vi "FormatCrvNames.vi"(8 "entrée d'erreur":errorcluster, 11 "CurveNamesIn":string[](array[string])) -> (0 "sortie d'erreur":errorcluster, 3 "CurveNames":string[](array[string]))   [LabVIEW 2019]
doc: "Ce Vi prend le tableau des noms de courbe au format Scanlist et retire la partie \"_Scan|Log\". La partie retiré correspond au caractère \"_\" suivi du préfixe de scan ou de log spécifié dans Labscan.ini. Pour les scan à plusieurs ordres, la partie spécifiant l'indice du paramètre de 2e ordre (ex: _par0) est remis en place.\nEx:\nTools.Temps Abs (ms)_Scan0 -> Tools.Temps Abs (ms)\nTools.Temps Abs (ms)_Scan0@Tools.Indice de Points(points)_par0 -> Tools.Temps Abs (ms)_par0"
uses:
  <vilib>/regexp/Match Regular Expression.xnode
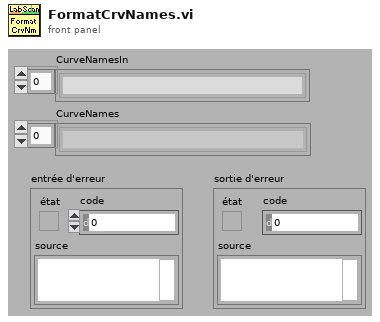
[diagram p1: front panel]
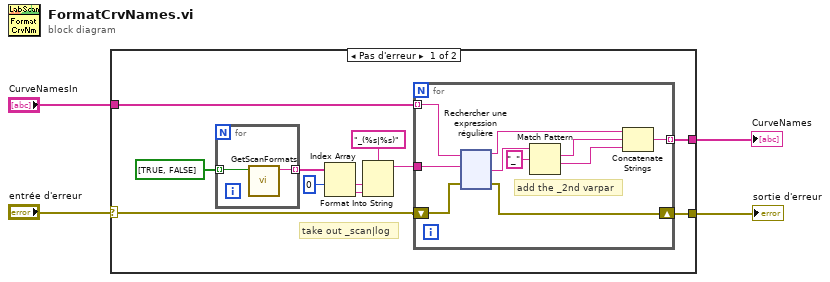
[diagram p0: block diagram]
diagram:
  n1 = case shown="Pas d'erreur" "entrée d'erreur" {
    selector: "entrée d'erreur" -> [w5 w139]
    tunnel: "CurveNamesIn" -> [w15 _]
    tunnel: [w7 _] -> w2
    tunnel: [w6 w139] -> w3
    frame No Error {
      # "take out _scan|log"
      n2 = for {
        tunnel: bool[] [TRUE, FALSE] -> [w138] mode=indexing
        tunnel: [w137] -> w13 mode=indexing
        n3 = call "GetScanFormats.vi"("Scan(T)"=w138) -> ("Prefixe"=w137:string)  [unwired: 8 in, 2 out]
      }
      n4 = Index Array(array=w13, index #1=0 ("indice")) -> (element #1=w10:string, element #2=w9:string)  [unwired: 1 in]
      n5 = Format Into String(format string="_(%s|%s)" ("chaîne de format"), w10, w9) -> (resulting string=w8:string)  [unwired: 2 in, 1 out]
      n6 = for {
        tunnel: w15 -> [w25] mode=indexing
        tunnel: w8 -> [w24]
        tunnel: [w20] -> w7 mode=indexing
        shift-right: [w17] -> w6
        shift-left: w5 -> [w16]
        # "add the _2nd varpar"
        n7 = xnode "Rechercher une expression régulière"("chaîne en entrée"=w25, "expression régulière"=w24, "entrée d'erreur"=w16) -> ("avant la correspondance"=w23:string, "après la correspondance"=w22:string, "sortie d'erreur"=w17:errorcluster)  [unwired: 3 in, 2 out]
        n8 = Match Pattern(string=w22, regular expression="_" ("expression régulière")) -> (match substring=w19:string, after substring=w18:string)  [unwired: 1 in, 2 out]
        n9 = Concatenate Strings(w23, w19, w18) -> (w20:string)
      }
    }
    frame Error {
    }
  }
  "sortie d'erreur" <- w3
  "CurveNames" <- w2
